vi "setColor.vi"(8 "Error In":errorcluster, 10 "color":refnum<class "QColor.lvclass">, 11 "QBrush In":refnum<class "QBrush.lvclass">) -> (0 "Error Out":errorcluster, 3 "QBrush Out":refnum<class "QBrush.lvclass">)   [LabVIEW 2014, in "QBrush.lvclass"]
doc: "LabVIEW-specific documentation is not yet available. See <b>https://doc.qt.io/qt-5/qbrush.html#setColor</b>"
uses:
  QBrush.lvclass
  QColor/QColor.lvclass
  LQ Core/LQSerialData/LQSerialData.lvclass/LQSerialData.ctl
  LQ Core/LQ Core.lvlib
  LQ Core/LQSerialData/LQSerialData.lvclass
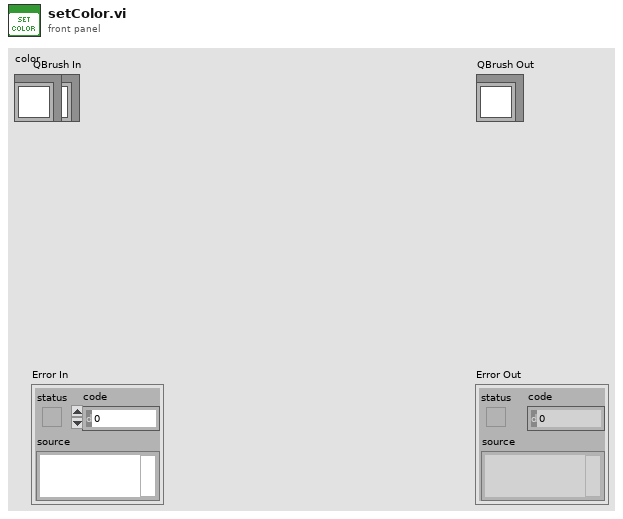
[diagram p1: front panel]
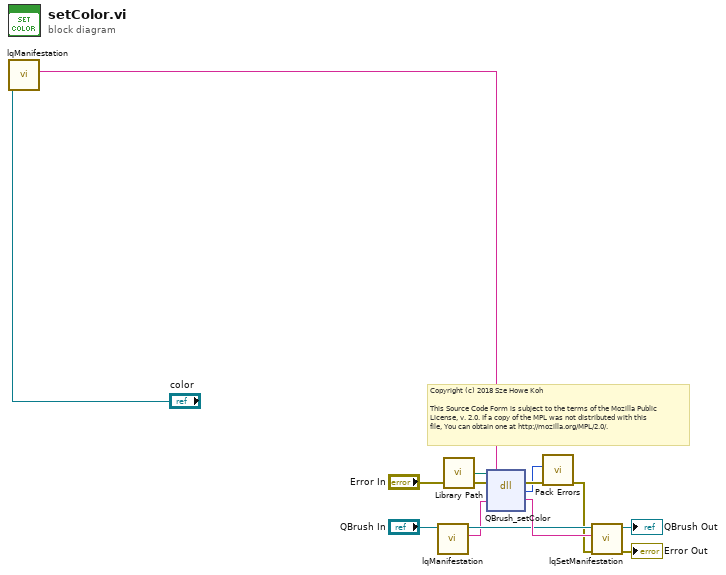
[diagram p0: block diagram]
diagram:
  # "Copyright (c) 2018 Sze Howe Koh\n\nThis Source Code Form is subject to the terms of the Mozilla Public\nLicense, v. 2.0. If a copy of the MPL was not distributed with this\nfile, You can obtain one at http://mozilla.org/MPL/2.0/."
  n1 = call "lqManifestation.vi"("LQSerialData in"="color") -> ("Manifestation"=w1:string)  [unwired: 9 in, 1 out]
  n2 = call "lqManifestation.vi"("LQSerialData in"="QBrush In") -> ("Manifestation"=w8:string, "LQSerialData out"=w9:refnum<class "QBrush.lvclass">)  [unwired: 9 in]
  n3 = call "Library Path.vi"() -> ("Library Path"=w7:path)
  n4 = dll-call lib="?" fn="QBrush_setColor"(path in=w7, error in="Error In", "_instance"=w8, "color"=w1) -> (error out=w6:errorcluster, w5:i32, "_instance"=w11:string)  [unwired: 2 in, 1 out]
  n5 = call "Pack Errors.vi"("Error In"=w6, "Error Code"=w5) -> ("Error Out"=w4:errorcluster)  [unwired: 9 in]
  n6 = call "lqSetManifestation.vi"("Error In"=w4, "Manifestation"=w11, "LQSerialData in"=w9) -> ("Error Out"=→"Error Out":errorcluster, "LQSerialData out"=→"QBrush Out":refnum<class "QBrush.lvclass">)  [unwired: 7 in]
